vi "Set - wForms.vi"(0 "reference in":refnum<class "GSwFormDSP.lvclass">, 5 "error in (no error)":errorcluster, 6 "Init wForms":bool, 7 "wForms":waveform(dbl)[](array[waveform])) -> (14 "reference out":refnum<class "GSwFormDSP.lvclass">, 19 "error out":errorcluster)   [LabVIEW 2022 SP3, in "GSwFormDSP.lvclass"]
uses:
  GSwFormDSP.lvclass
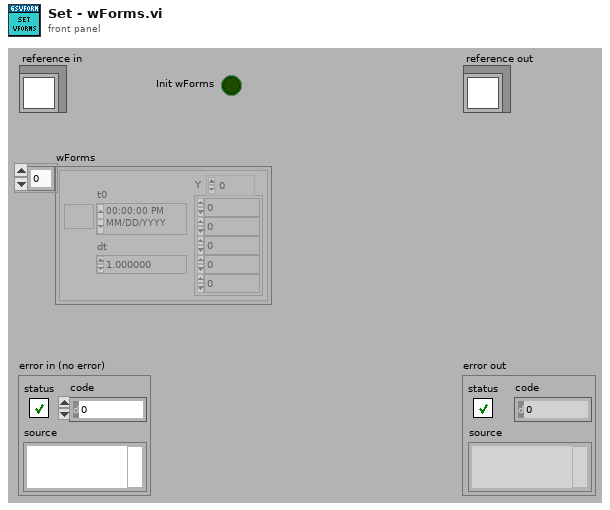
[diagram p1: front panel]
types:
  T1 = typedef "GSwFormDSP.lvclass/ObjectAttributesRef.ctl" = refnum<data-value>
  T2 = typedef "GSwFormDSP.lvclass/ObjectAttributes.ctl" = cluster{"Wform Ref":refnum<data-value>, "Nb Signals":i32, "Spectral Function Parameters":T3, "FFT":waveform(cdb)[], "Nb FFT":i32, "Nb Averages":i32[], "Reference Indexes":i32[], "Response Indexes":i32[], "Coherence":waveform(dbl)[], "TDF Parameters":T5, "DAQ":cluster{"Duration (sec)":dbl, "Buffer Size (Samples)":i32, "Offset (Samples)":i32}, "Filter Impulse Response (TDF)":waveform(dbl), "Sound Playback":T6}
  T3 = typedef "GSwFormDSP.lvclass/Spectral Parameters.ctl" = cluster{"Frequency resolution (Hz)":dbl, "Overlap":dbl, "Window":T4}
  T4 = typedef "NI_AALPro.lvlib/windowTd.ctl" = u32
  T5 = typedef "GSwFormDSP.lvclass/TDF Parameters.ctl" = cluster{"Filter":enum32{"Lowpass", "Highpass", "Bandpass", "Bandstop"}, "Type:":enum16{"Butterworth", "Chebyshev", "Inv Chebyshev", "Elliptic", "Bessel"}, "LP cutoff freq":dbl, "HP cutoff freq":dbl, "Order":i32, "passband ripple (dB)":dbl, "stopband attenuation (dB)":dbl, "Phaseless Filter":bool, "Include Fade IN and OUT":bool}
  T6 = typedef "GSwFormDSP.lvclass/Sound Playback.ctl" = cluster{"Timer start (ms)":u32, "task ID":T7, "Cursor Init Location (s)":dbl, "SC Volume":dbl}
  T7 = typedef "Sound Output Task ID.ctl" = u32
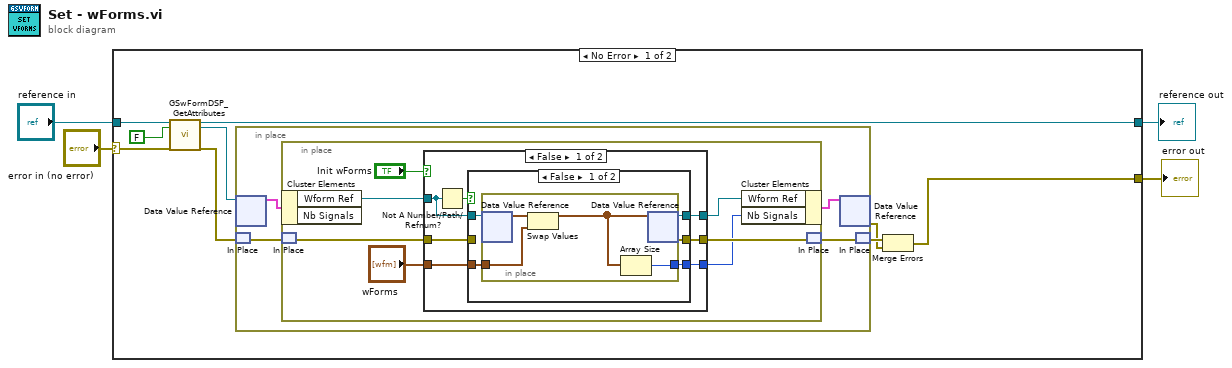
[diagram p0: block diagram]
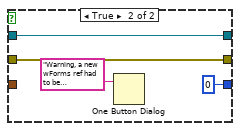
[diagram p2: hidden frame]
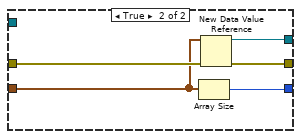
[diagram p3: hidden frame]
diagram:
  n1 = case shown="No Error" "error in (no error)" {
    selector: "error in (no error)" -> [w11 w51]
    tunnel: [w5 w51] -> w3
    tunnel: [w8 w50] -> w1
    tunnel: "reference in" -> [w13 w50]
    frame No Error {
      n2 = call "GSwFormDSP_GetAttributes.vi"("reference in"=w13, "return data? (T)"=FALSE, "error in (no error)"=w11) -> ("reference out"=w8:refnum<class "GSwFormDSP.lvclass">, "attributes ref"=w10:T1, "error out"=w9:errorcluster)  [unwired: 13 in, 1 out]
      n3 = in-place {
        n4 = in-place-dvr #1(w10) -> (w16:T2)  [unwired: 1 out]
        n5 = in-place-match #2(w9) -> (w15:errorcluster)
        n6 = in-place {
          n7 = in-place-cluster #3(w16) -> ("Wform Ref"=w22:refnum<data-value>)  [unwired: 1 out]
          n8 = in-place-match #4(w15) -> (w23:errorcluster)
          n9 = case shown="False" "Init wForms" {
            tunnel: w22 -> [w27 _]
            tunnel: w23 -> [w25 w49]
            tunnel: [w29 w48] -> w21
            tunnel: [w31 w47] -> w20
            tunnel: "wForms" -> [w30 w46]
            tunnel: [w28 w45] -> w19
            frame False {
              n10 = Not A Number/Path/Refnum?(number/path/refnum=w27) -> (NaN/Path/Refnum?=w26:bool)
              n11 = case shown="False" w26 {
                tunnel: [w36 w42] -> w31
                tunnel: w30 -> [w35 _]
                tunnel: [w34 w44] -> w29
                tunnel: [w33 0] -> w28
                tunnel: w27 -> [w32 w42]
                tunnel: w25 -> [_ w44]
                frame False {
                  n12 = in-place {
                    in-place-border: w35 -> [w39]
                    in-place-border: [w37] -> w33
                    n13 = in-place-dvr #5(w32) -> (w40:waveform(dbl)[])  [unwired: 1 out]
                    n14 = Swap Values(12:w40, 14:w39) -> (1:w38:waveform(dbl)[])  [unwired: 1 in, 1 out]
                    n15 = Array Size(array=w38) -> (size(s)=w37:i32)
                    n16 = in-place-dvr #5(w38) -> (w36:refnum<data-value>, w34:errorcluster)
                  }
                }
                frame True {
                  n17 = One Button Dialog(message="Warning, a new wForms ref had to be created???") -> ()  [unwired: 1 in, 1 out]
                }
              }
            }
            frame True {
              n18 = Array Size(array=w46) -> (size(s)=w45:i32)
              n19 = New Data Value Reference(data value=w46, error in=w49) -> (data value reference=w47:refnum<data-value>, error out=w48:errorcluster)
            }
          }
          n20 = in-place-cluster #3("Wform Ref"=w20, "Nb Signals"=w19) -> (w17:T2)
          n21 = in-place-match #4(w21) -> (w14:errorcluster)
        }
        n22 = in-place-dvr #1(w17) -> (w6:errorcluster)  [unwired: 1 out]
        n23 = in-place-match #2(w14) -> (w7:errorcluster)
      }
      n24 = Merge Errors(w7, w6) -> (w5:errorcluster)
    }
    frame Error {
    }
  }
  "error out" <- w3
  "reference out" <- w1
